vi "exercise2.vi"() -> ()   [LabVIEW 2021]
panel:
  in  "stop":bool
  out "Received Value 2":dbl
  out "Received Value 1":dbl
  out "String that is Received":string
  out "bytes written":i32
  out "string that is sent":string
  in  "Send Value 2":dbl
  in  "Send Value 1":dbl
  in  "send Button":bool
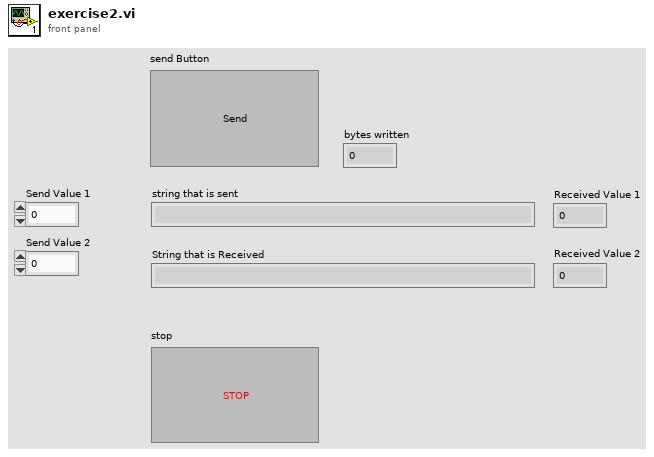
[diagram p1: front panel]
types:
  T1 = enum16{"Standard", "Buffered", "CRLF", "Immediate"}
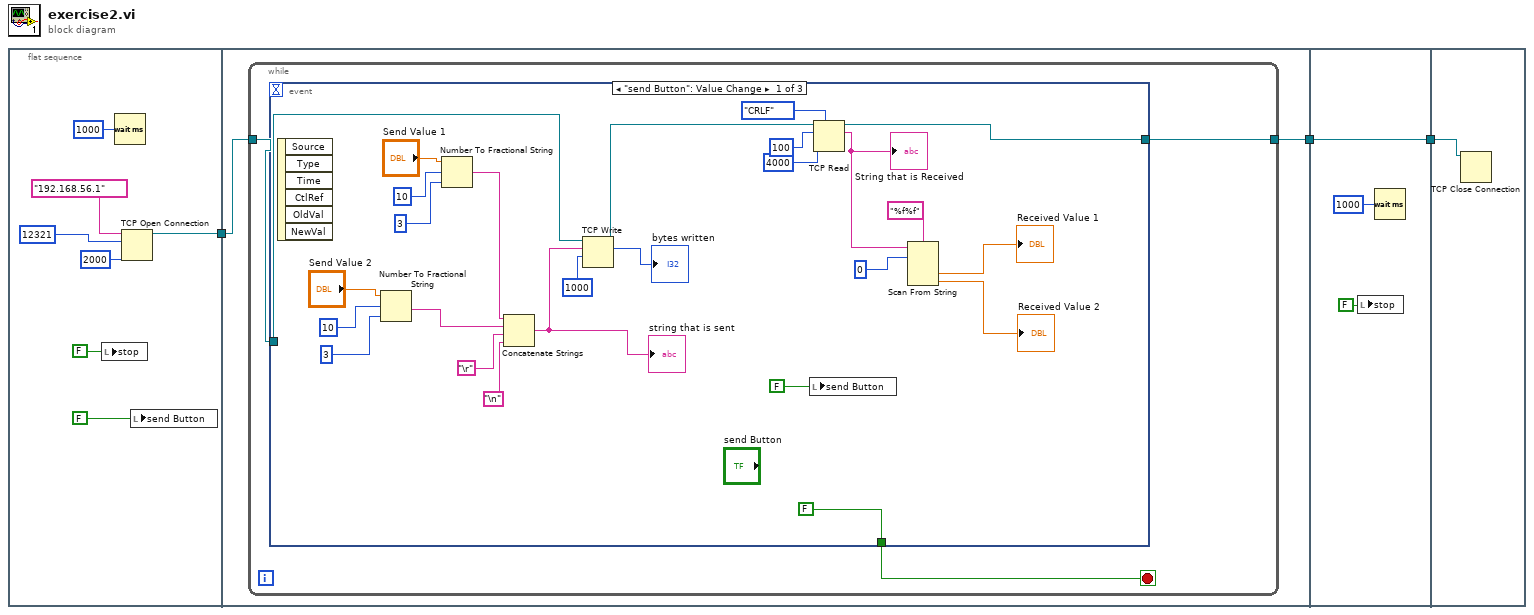
[diagram p0: block diagram]
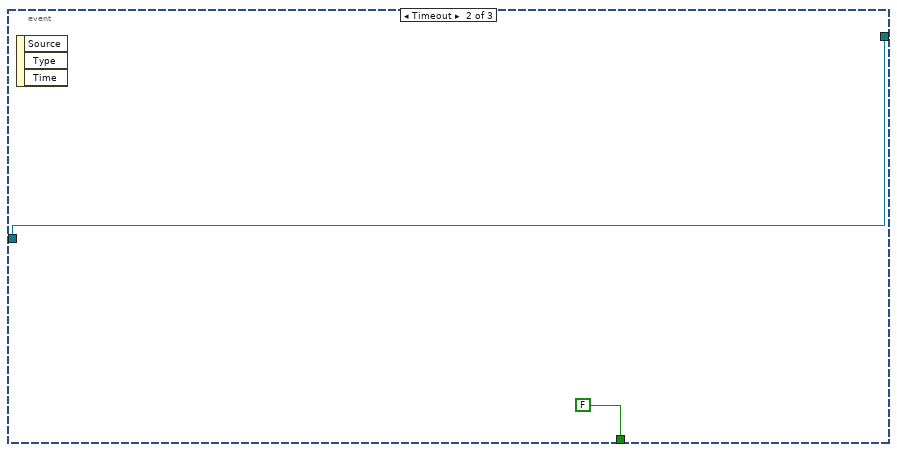
[diagram p2: hidden frame]
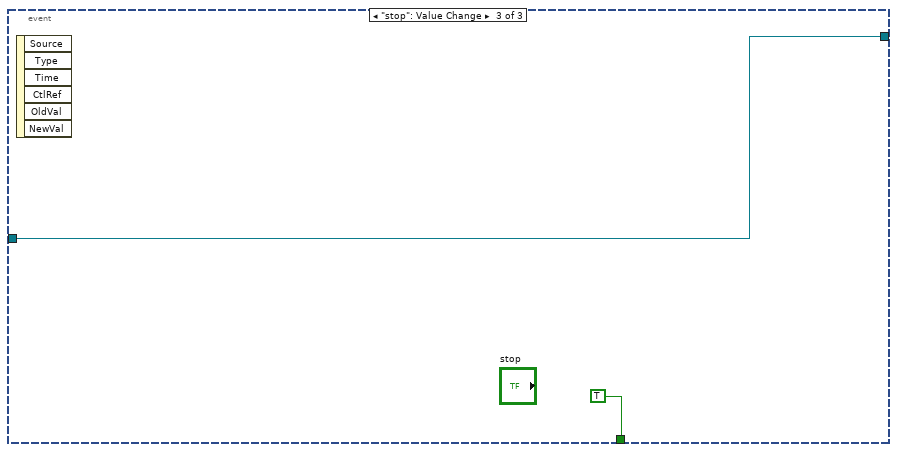
[diagram p3: hidden frame]
diagram:
  n1 = flat-sequence {
    tunnel: [w4] -> w3
    tunnel: w3 -> [w12]
    tunnel: [w11] -> w2
    tunnel: w2 -> [w48]
    tunnel: [w48] -> w1
    tunnel: w1 -> [w49]
    frame #0 {
      n2 = local write "stop"(FALSE) -> ()
      n3 = Wait (ms)(milliseconds to wait=u32 1000) -> ()  [unwired: 1 out]
      n4 = TCP Open Connection(address="192.168.56.1", remote port or service name=u16 12321, timeout ms (60000)=2000) -> (connection ID=w4:refnum<k5>)  [unwired: 2 in, 1 out]
      n5 = local write "send Button"(FALSE) -> ()
    }
    frame #1 {
      n6 = while {
        tunnel: w12 -> [w15]
        tunnel: [w14] -> w11
        stop <- w13 stop-if-true
        n7 = event shown="[0] \"send Button\": Value Change" {
          selector: _ -> [_ _ _]
          dyn-events: _ -> [_ _ _]
          timeout: _ -> [_ _ _]
          tunnel: w15 -> [w16 w43 w45]
          tunnel: [w21 w43 w45] -> w14
          tunnel: [FALSE FALSE TRUE] -> w13
          event "send Button": Value Change {
            n8 = event-data() -> ()  [unwired: 1 in, 6 out]
            n9 = Number To Fractional String(number="Send Value 2", width (-)=10, precision (6)=3) -> (F-format string=w32:string)  [unwired: 1 in]
            n10 = Number To Fractional String(number="Send Value 1", width (-)=10, precision (6)=3) -> (F-format string=w31:string)  [unwired: 1 in]
            n11 = Concatenate Strings(w31, w32, "\r", "\n") -> (w33:string)
            "string that is sent" <- w33
            n12 = TCP Write(connection ID=w16, data in=w33, 9:1000 ("timeout ms (25000)")) -> (connection ID out=w17:refnum<k5>, bytes written=→"bytes written":i32)  [unwired: 1 in, 1 out]
            n13 = local write "send Button"(FALSE) -> ()
            n14 = TCP Read(connection ID=w17, bytes to read=100, 7:T1."CRLF" ("mode (standard)"), 9:4000 ("timeout ms (25000)")) -> (connection ID out=w21:refnum<k5>, data out=w26:string)  [unwired: 1 in, 1 out]
            "String that is Received" <- w26
            n15 = Scan From String(format string="%f%f", input string=w26, initial scan location=u32 0) -> (output 1=→"Received Value 1":dbl, output 2=→"Received Value 2":dbl)  [unwired: 3 in, 3 out]
          }
          event Timeout {
            n16 = event-data() -> ()  [unwired: 1 in, 3 out]
          }
          event "stop": Value Change {
            n17 = event-data() -> ()  [unwired: 1 in, 6 out]
          }
        }
      }
    }
    frame #2 {
      n18 = local write "stop"(FALSE) -> ()
      n19 = Wait (ms)(milliseconds to wait=u32 1000) -> ()  [unwired: 1 out]
    }
    frame #3 {
      n20 = TCP Close Connection(connection ID=w49) -> ()  [unwired: 2 in, 2 out]
    }
  }
